vi "HDF5_Init_Disdrometer_Refs.vi"(5 "HDF5 file ref":T2 format="%.0x", 9 "File Exists?":bool, 11 "error in":errorcluster) -> (4 "DisdromRefs":T1 {"Status_dset_deprecated" format="%.0x"; "Spectrum_dset" format="%.0x"; "SpectGroup_ref" format="%.0x"; "HydromType_dset" format="%.0x"; "UnknownVolum_dset" format="%.0x"; "UnknownParticls_dset" format="%.0x"; "NonHydrVolum_dset" format="%.0x"; "NonHydrParticls_dset" format="%.0x"; "ParticlMinDiam_dset" format="%.0x"; "ParticlMaxSpeed_dset" format="%.0x"; "RadarReflect_dset" format="%.0x"; "Visibility_dset" format="%.0x"; "TotalRain_dset" format="%.0x"; "Solid_dset" format="%.0x"; "Liquid_dset" format="%.0x"; "TotalRainRate_dset" format="%.0x"; "TimeStamp_dset" format="%.0x"; "ParticlMinSpeed_dset" format="%.0x"; "MeasdParticles_dset" format="%.0x"; "MaxDiam_dset" format="%.0x"; "BasicGroup_ref" format="%.0x"}, 15 "error out":errorcluster)   [LabVIEW 2018]
doc: "Set up the HDF5 data structure and initialize the references for the Noise1, Noise2, Noise3, and Noise4 Datasets (tables).\n\nData structure:\nNoise1 (Dataset) - 1024 element Double array (waveform) \nNoise2 (Dataset) - 1024 element Double array (waveform) \nNoise3 (Dataset) - 1024 element Double array (waveform) \nNoise4 (Dataset) - 1024 element Double array (waveform)"
uses:
  <vilib>/addons/h5labview2/base/hid_t.ctl
  HDF5_Disdrometer_Refs.ctl
  DisdrometerData.ctl
  DisdromterSummaryData.ctl
  Disdrometer/Disdrometer_Status_Cluster.ctl
  lib_path_mod_20200519.vi
  <vilib>/addons/h5labview2/base/H5Equery.vi
  <vilib>/addons/h5labview2/attrib/H5Awrite.llb/H5Awrite.xnode
  <vilib>/addons/h5labview2/group/H5G.lvlib
  <vilib>/addons/h5labview2/dataset/H5D.lvlib
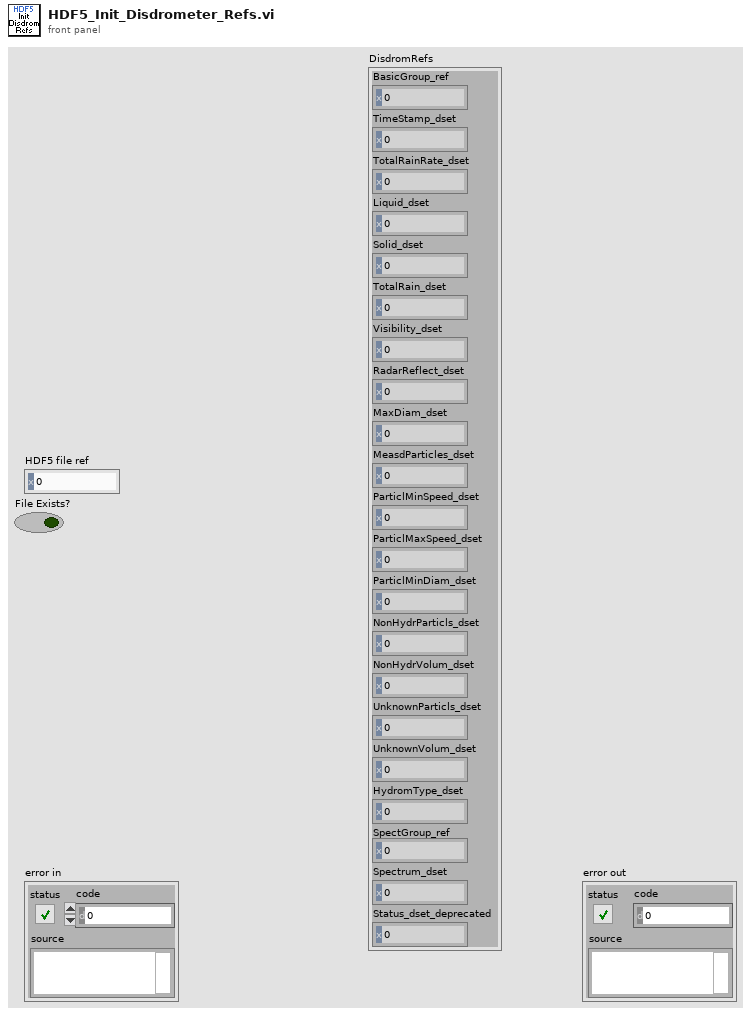
[diagram p1: front panel]
types:
  T1 = typedef "HDF5_Disdrometer_Refs.ctl" = cluster{"BasicGroup_ref":T2, "TimeStamp_dset":T2, "TotalRainRate_dset":T2, "Liquid_dset":T2, "Solid_dset":T2, "TotalRain_dset":T2, "Visibility_dset":T2, "RadarReflect_dset":T2, "MaxDiam_dset":T2, "MeasdParticles_dset":T2, "ParticlMinSpeed_dset":T2, "ParticlMaxSpeed_dset":T2, "ParticlMinDiam_dset":T2, "NonHydrParticls_dset":T2, "NonHydrVolum_dset":T2, "UnknownParticls_dset":T2, "UnknownVolum_dset":T2, "HydromType_dset":T2, "SpectGroup_ref":T2, "Spectrum_dset":T2, "Status_dset_deprecated":T2}
  T2 = typedef "hid_t.ctl" = i32
  T3 = typedef "DisdrometerData.ctl" = cluster{"Spectrum Data":i16[], "DisdromSummary":T4, "Status":T5}
  T4 = typedef "DisdromterSummaryData.ctl" = cluster{"current time":dbl, "Timestamp":dbl, "Total Rain Rate":dbl, "Liquid Rain Rate":dbl, "Solid Rain Rate":dbl, "Total Rainfall":dbl, "Visibility":dbl, "Radar Reflectivity":dbl, "Max Diameter Hail":dbl, "Measured Particles":i32, "Particle Min Speed":i16, "Particle Max Speed":i16, "Particle Min Diam":i16, "NonHydr Particles":i16, "NonHydr Volume":dbl, "Unkn Particles":i16, "Unkn Volume":dbl, "HydroType":i8}
  T5 = typedef "Disdrometer_Status_Cluster.ctl" = cluster{"Laser":bool, "Signal":bool, "LaserTemp_Analog":bool, "LaserTemp_Digital":bool, "LaserCurrent_Analog":bool, "LaserCurrent_Digital":bool, "SensorSupply":bool, "HeatLaserHead":bool, "HeatReceiverHead":bool, "TempSensor":bool, "HeatSupply":bool, "HeatHousing":bool, "HeatHeads":bool, "HeatCarriers":bool, "OutputLaserPower":bool, "Checksum":bool, "StatusInt":u16}
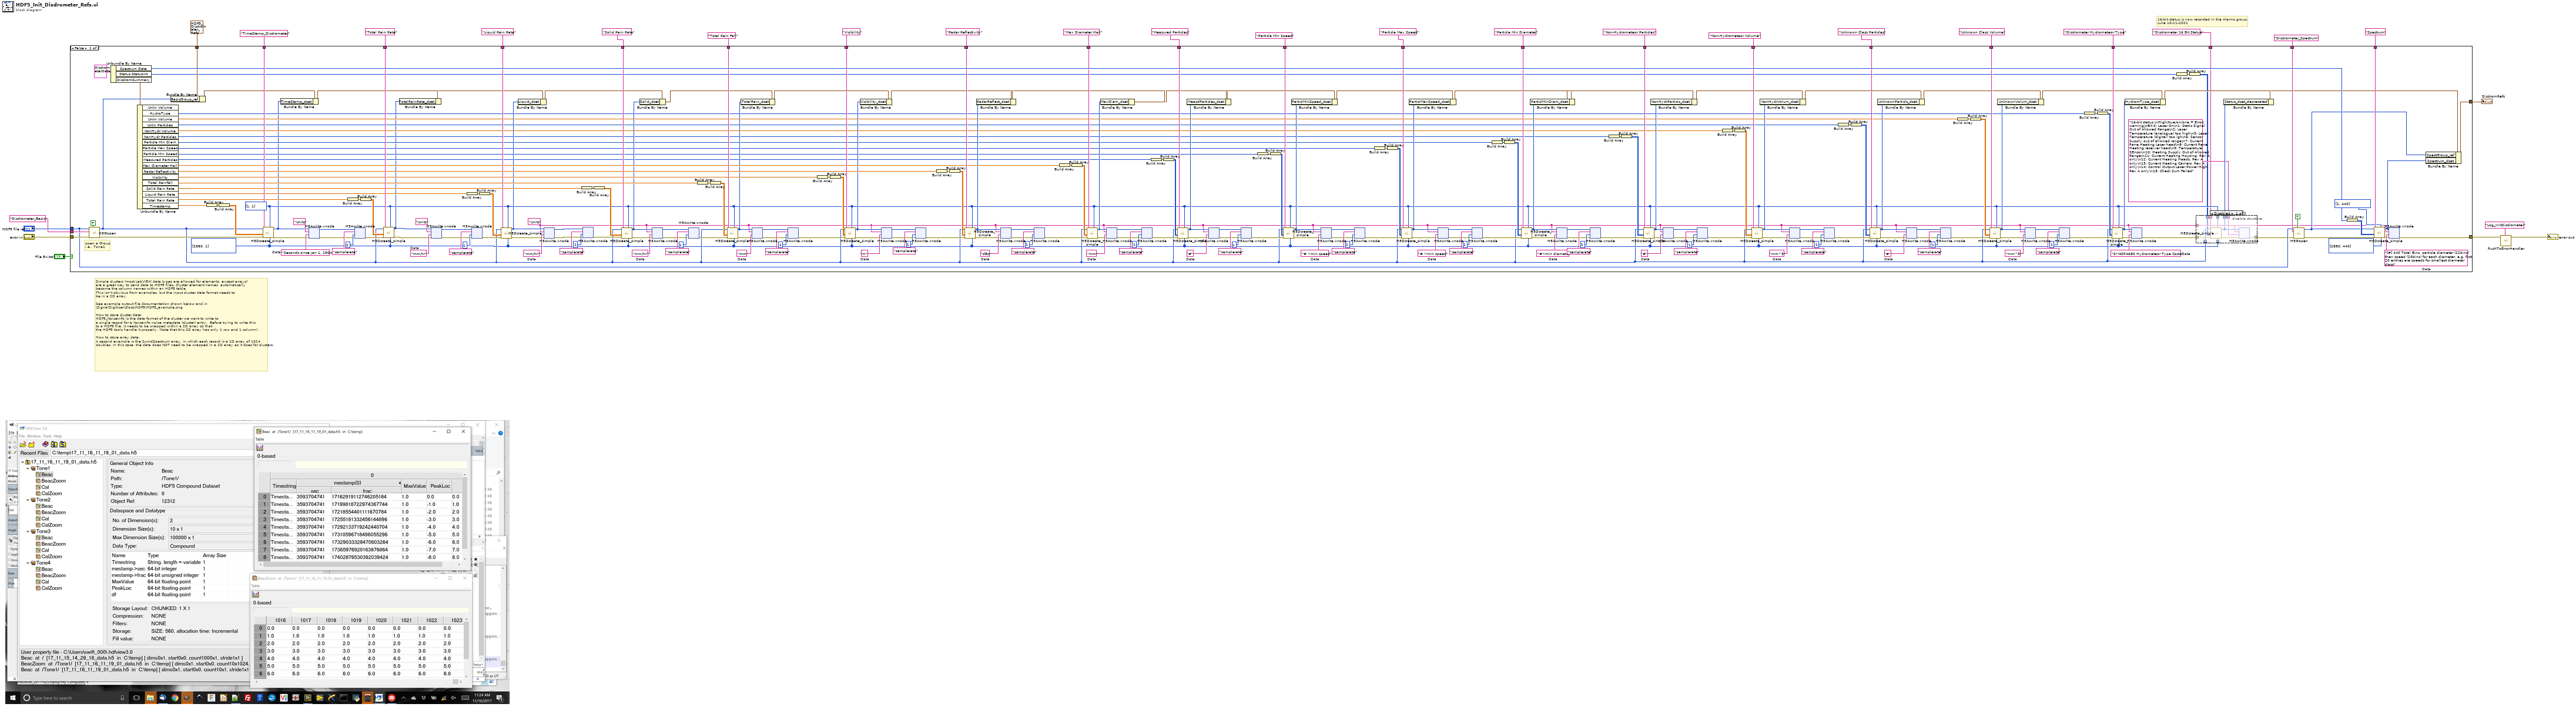
[diagram p0: block diagram]
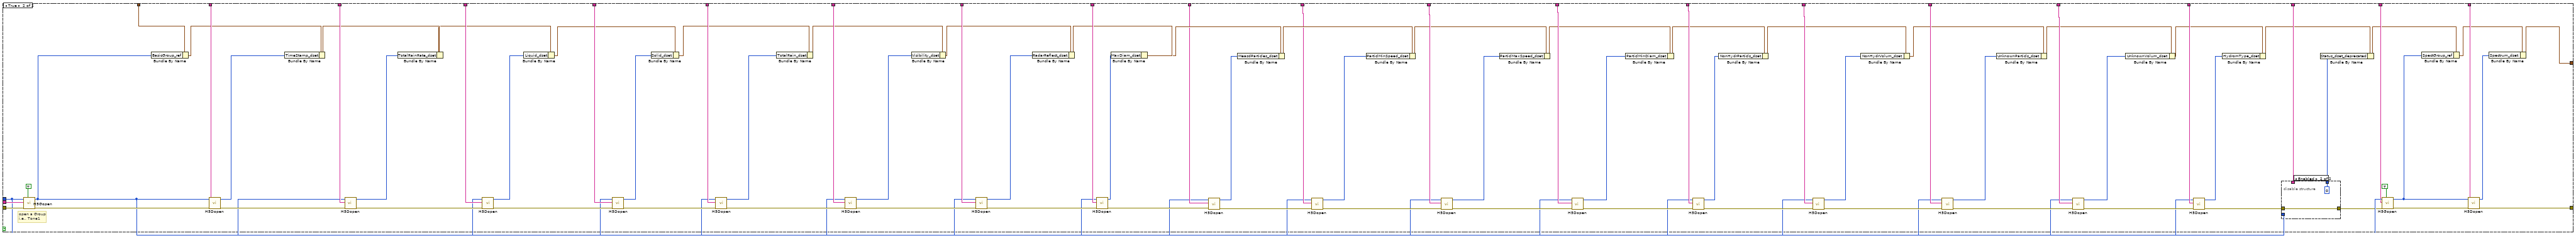
[diagram p3: hidden frame]
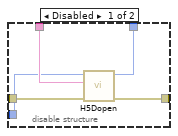
[diagram p4: hidden frame]
diagram:
  # "16-bit status is now recorded in the Alarms group.\nLuke 10-11-2021"
  # "Simple clusters (most LabVIEW data types are allowed for elements, except arrays) \nare a great way to send data to HDF5 files. Cluster element names  automatically\nbecome the column names within an HDF5 table.\nThis isn't obvious from examples, but the input cluster data format needs to \nbe in a 2D array.\n\nSee example output file documentation shown below and in\n\\SignalDigitizer\\Docs\\HDF5\\HDF5_example.png\n\nHow to store cluster data:\nHDF5_NoiseInfo is the data format of the cluster we want to write to \na single record for a NoiseInfo noise metadata (cluster) entry.  Before trying to write this \nto a HDF5 file, it needs to be wrapped within a 2D array so that \nthe HDF5 tools handle it properly. (Note that this 2D array has only 1 row and 1 column).\n\nHow to store array data:\nA second example is the SumdSpectrum array, in which each record is a 1D array of 1024 \ndoubles. In this case, the data does NOT need to be wrapped in a 2D array as it does for clusters."
  n1 = case shown="False" "File Exists?" {
    tunnel: "error in" -> [w283 w1049]
    tunnel: "HDF5 file ref" -> [w178 w1006]
    tunnel: T1 {"BasicGroup_ref"=0, "TimeStamp_dset"=0, "TotalRainRate_dset"=0, "Liquid_dset"=0, "Solid_dset"=0, "TotalRain_dset"=0, "Visibility_dset"=0, "RadarReflect_dset"=0, "MaxDiam_dset"=0, "MeasdParticles_dset"=0, "ParticlMinSpeed_dset"=0, "ParticlMaxSpeed_dset"=0, "ParticlMinDiam_dset"=0, "NonHydrParticls_dset"=0, "NonHydrVolum_dset"=0, "UnknownParticls_dset"=0, "UnknownVolum_dset"=0, "HydromType_dset"=0, "SpectGroup_ref"=0, "Spectrum_dset"=0, "Status_dset_deprecated"=0} ("Cluster") -> [w269 w1029]
    tunnel: "TimeStamp_Disdrometer" ("string") -> [w278 w1046]
    tunnel: "Disdrometer_Basic" ("name") -> [w277 w1045]
    tunnel: [w276 w1010] -> w24
    tunnel: "Spectrum" ("string") -> [w273 w1044]
    tunnel: "Total Rain Rate" ("string") -> [w265 w1037]
    tunnel: "Liquid Rain Rate" ("string") -> [w257 w1038]
    tunnel: "Solid Rain Rate" ("string") -> [w252 w1039]
    tunnel: "Total Rain Fall" ("string") -> [w249 w1040]
    tunnel: "Visibility" ("string") -> [w241 w1041]
    tunnel: "Radar Reflectivity" ("string") -> [w237 w1042]
    tunnel: "Max Diameter Hail" ("string") -> [w232 w1043]
    tunnel: [w213 w1009] -> w4
    tunnel: "Disdrometer_Spectrum" ("name") -> [w211 w1005]
    tunnel: "Measured Particles" ("string") -> [w183 w997]
    tunnel: "Particle Min Speed" ("string") -> [w186 w991]
    tunnel: "Particle Max Speed" ("string") -> [w191 w990]
    tunnel: "Particle Min Diameter" ("string") -> [w194 w989]
    tunnel: "Non-Hydrometeor Particles" ("string") -> [w198 w988]
    tunnel: "Non-Hydrometeor Volume" ("string") -> [w172 w976]
    tunnel: "Unknown Class Particles" ("string") -> [w168 w975]
    tunnel: "Unknown Class Volume" ("string") -> [w165 w974]
    tunnel: "Disdrometer Hydrometeor Type" ("string") -> [w161 w973]
    tunnel: "Disdrometer 16 Bit Status" ("string") -> [w32 w965]
    frame False {
      w138 = "Seconds since Jan 1, 1904"  # Data
      w139 = "mm/hr"  # Data
      w153 = "SYNOP4680 Hydrometeor Type Code"  # Data
      w157 = "mm^3"  # Data
      w158 = "#"  # Data
      w159 = "mm^3"  # Data
      w209 = "#"  # Data
      w203 = "#<min diameter"  # Data
      w202 = "# >min speed"  # Data
      w201 = "# <min speed"  # Data
      w200 = "#"  # Data
      w217 = "[#] 440 Total Bins, particle diameter (22bins) then speed (20bins) for each diameter, e.g. first 20 entries are speeds for smallest diameter class"  # Data
      w218 = "mm"  # Data
      w224 = "dBz"  # Data
      w225 = "m"  # Data
      w226 = "mm"  # Data
      w227 = "mm/hr"  # Data
      w35 = "Units" ("attrib name")
      w230 = "mm/hr"  # Data
      w43 = i32[] [1, 1] ("size(s)")
      w30 = u64[] [2880, 1] ("max size")
      # "open a Group\ni.e., Tone1"
      n2 = call <vilib>:"H5Gopen.vi"("create? (F)"=TRUE, "error in (no error)"=w283, "name"=w277, "ref in"=w178) -> ("error out"=w279:errorcluster, "group out"=w42:T2)  [unwired: 6 in]
      n3 = Unbundle By Name(T3 {"Spectrum Data"=[], "DisdromSummary"={"current time"=0.0, "Timestamp"=0.0, "Total Rain Rate"=0.0, "Liquid Rain Rate"=0.0, "Solid Rain Rate"=0.0, "Total Rainfall"=0.0, "Visibility"=0.0, "Radar Reflectivity"=0.0, "Max Diameter Hail"=0.0, "Measured Particles"=0, "Particle Min Speed"=0, "Particle Max Speed"=0, "Particle Min Diam"=0, "NonHydr Particles"=0, "NonHydr Volume"=0.0, "Unkn Particles"=0, "Unkn Volume"=0.0, "HydroType"=0}, "Status"={"Laser"=TRUE, "Signal"=TRUE, "LaserTemp_Analog"=TRUE, "LaserTemp_Digital"=TRUE, "LaserCurrent_Analog"=TRUE, "LaserCurrent_Digital"=TRUE, "SensorSupply"=TRUE, "HeatLaserHead"=TRUE, "HeatReceiverHead"=TRUE, "TempSensor"=TRUE, "HeatSupply"=TRUE, "HeatHousing"=TRUE, "HeatHeads"=TRUE, "HeatCarriers"=TRUE, "OutputLaserPower"=TRUE, "Checksum"=TRUE, "StatusInt"=0}}) -> ("Spectrum Data"=w272:i16[], "Status.StatusInt"=w31:u16, "DisdromSummary"=w263:T4)
      n4 = Unbundle By Name(w263) -> ("HydroType"=w141:i8, "Unkn Volume"=w142:dbl, "Unkn Particles"=w143:i16, "NonHydr Volume"=w144:dbl, "NonHydr Particles"=w145:i16, "Particle Min Diam"=w146:i16, "Particle Max Speed"=w147:i16, "Particle Min Speed"=w148:i16, "Measured Particles"=w149:i32, "Max Diameter Hail"=w233:dbl, "Radar Reflectivity"=w238:dbl, "Visibility"=w243:dbl, "Total Rainfall"=w248:dbl, "Solid Rain Rate"=w253:dbl, "Liquid Rain Rate"=w258:dbl, "Total Rain Rate"=w261:dbl, "Timestamp"=w262:dbl)  [unwired: 1 out]
      n5 = Bundle By Name(cluster=w269, "BasicGroup_ref"=w42) -> (w268:T1)
      n6 = Build Array(w262) -> (w282:dbl[])
      n7 = Build Array(w282) -> (w281:dbl[][])
      n8 = call <vilib>:"H5Dcreate_simple.vi"("max size"=w30, "chunk size"=w43, "error in (no error)"=w279, "type in"=w281, "name"=w278, "ref in"=w42) -> ("error out"=w136:errorcluster, "dset out"=w133:T2)  [unwired: 4 in]
      n9 = Bundle By Name(cluster=w268, "TimeStamp_dset"=w133) -> (w264:T1)
      n10 = xnode "H5Awrite.xnode"("error in (no error)"=w136, "data"=w138, "attrib name"="Units", "ref in"=w133) -> ("error out"=w121:errorcluster, "ref out"=w119:i32)  [unwired: 3 in, 1 out]
      n11 = Build Array(w261) -> (w266:dbl[])
      n12 = xnode "H5Awrite.xnode"("error in (no error)"=w121, "data"=u32 1, "attrib name"="samplerate", "ref in"=w119) -> ("error out"=w120:errorcluster)  [unwired: 3 in, 2 out]
      n13 = Build Array(w266) -> (w267:dbl[][])
      n14 = call <vilib>:"H5Dcreate_simple.vi"("max size"=w30, "chunk size"=w43, "error in (no error)"=w120, "type in"=w267, "name"=w265, "ref in"=w42) -> ("error out"=w135:errorcluster, "dset out"=w134:T2)  [unwired: 4 in]
      n15 = Bundle By Name(cluster=w264, "TotalRainRate_dset"=w134) -> (w256:T1)
      n16 = xnode "H5Awrite.xnode"("error in (no error)"=w135, "data"=w139, "attrib name"="Units", "ref in"=w134) -> ("error out"=w116:errorcluster, "ref out"=w114:i32)  [unwired: 3 in, 1 out]
      n17 = Build Array(w258) -> (w260:dbl[])
      n18 = xnode "H5Awrite.xnode"("error in (no error)"=w116, "data"=u32 1, "attrib name"="samplerate", "ref in"=w114) -> ("error out"=w115:errorcluster)  [unwired: 3 in, 2 out]
      n19 = Build Array(w260) -> (w259:dbl[][])
      n20 = call <vilib>:"H5Dcreate_simple.vi"("max size"=w30, "chunk size"=w43, "error in (no error)"=w115, "type in"=w259, "name"=w257, "ref in"=w42) -> ("error out"=w229:errorcluster, "dset out"=w228:T2)  [unwired: 4 in]
      n21 = Bundle By Name(cluster=w256, "Liquid_dset"=w228) -> (w247:T1)
      n22 = xnode "H5Awrite.xnode"("error in (no error)"=w229, "data"=w230, "attrib name"=w35, "ref in"=w228) -> ("error out"=w111:errorcluster, "ref out"=w110:i32)  [unwired: 3 in, 1 out]
      n23 = Build Array(w253) -> (w254:dbl[])
      n24 = xnode "H5Awrite.xnode"("error in (no error)"=w111, "data"=u32 1, "attrib name"="samplerate", "ref in"=w110) -> ("error out"=w109:errorcluster)  [unwired: 3 in, 2 out]
      n25 = Build Array(w254) -> (w255:dbl[][])
      n26 = call <vilib>:"H5Dcreate_simple.vi"("max size"=w30, "chunk size"=w43, "error in (no error)"=w109, "type in"=w255, "name"=w252, "ref in"=w42) -> ("error out"=w222:errorcluster, "dset out"=w223:T2)  [unwired: 4 in]
      n27 = Bundle By Name(cluster=w247, "Solid_dset"=w223) -> (w246:T1)
      n28 = xnode "H5Awrite.xnode"("error in (no error)"=w222, "data"=w227, "attrib name"=w35, "ref in"=w223) -> ("error out"=w106:errorcluster, "ref out"=w105:i32)  [unwired: 3 in, 1 out]
      n29 = xnode "H5Awrite.xnode"("error in (no error)"=w106, "data"=u32 1, "attrib name"="samplerate", "ref in"=w105) -> ("error out"=w104:errorcluster)  [unwired: 3 in, 2 out]
      n30 = Build Array(w248) -> (w251:dbl[])
      n31 = Build Array(w251) -> (w250:dbl[][])
      n32 = call <vilib>:"H5Dcreate_simple.vi"("max size"=w30, "chunk size"=w43, "error in (no error)"=w104, "type in"=w250, "name"=w249, "ref in"=w42) -> ("error out"=w129:errorcluster, "dset out"=w221:T2)  [unwired: 4 in]
      n33 = Bundle By Name(cluster=w246, "TotalRain_dset"=w221) -> (w242:T1)
      n34 = xnode "H5Awrite.xnode"("error in (no error)"=w129, "data"=w226, "attrib name"=w35, "ref in"=w221) -> ("error out"=w101:errorcluster, "ref out"=w100:i32)  [unwired: 3 in, 1 out]
      n35 = xnode "H5Awrite.xnode"("error in (no error)"=w101, "data"=u32 1, "attrib name"="samplerate", "ref in"=w100) -> ("error out"=w99:errorcluster)  [unwired: 3 in, 2 out]
      n36 = Build Array(w243) -> (w244:dbl[])
      n37 = Build Array(w244) -> (w245:dbl[][])
      n38 = call <vilib>:"H5Dcreate_simple.vi"("max size"=w30, "chunk size"=w43, "error in (no error)"=w99, "type in"=w245, "name"=w241, "ref in"=w42) -> ("error out"=w130:errorcluster, "dset out"=w220:T2)  [unwired: 4 in]
      n39 = Bundle By Name(cluster=w242, "Visibility_dset"=w220) -> (w236:T1)
      n40 = xnode "H5Awrite.xnode"("error in (no error)"=w130, "data"=w225, "attrib name"=w35, "ref in"=w220) -> ("error out"=w96:errorcluster, "ref out"=w95:i32)  [unwired: 3 in, 1 out]
      n41 = xnode "H5Awrite.xnode"("error in (no error)"=w96, "data"=u32 1, "attrib name"="samplerate", "ref in"=w95) -> ("error out"=w94:errorcluster)  [unwired: 3 in, 2 out]
      n42 = Build Array(w238) -> (w240:dbl[])
      n43 = Build Array(w240) -> (w239:dbl[][])
      n44 = call <vilib>:"H5Dcreate_simple.vi"("max size"=w30, "chunk size"=w43, "error in (no error)"=w94, "type in"=w239, "name"=w237, "ref in"=w42) -> ("error out"=w131:errorcluster, "dset out"=w219:T2)  [unwired: 4 in]
      n45 = Bundle By Name(cluster=w236, "RadarReflect_dset"=w219) -> (w231:T1)
      n46 = xnode "H5Awrite.xnode"("error in (no error)"=w131, "data"=w224, "attrib name"=w35, "ref in"=w219) -> ("error out"=w91:errorcluster, "ref out"=w90:i32)  [unwired: 3 in, 1 out]
      n47 = xnode "H5Awrite.xnode"("error in (no error)"=w91, "data"=u32 1, "attrib name"="samplerate", "ref in"=w90) -> ("error out"=w89:errorcluster)  [unwired: 3 in, 2 out]
      n48 = Build Array(w233) -> (w234:dbl[])
      n49 = Build Array(w234) -> (w235:dbl[][])
      n50 = call <vilib>:"H5Dcreate_simple.vi"("chunk size"=w43, "error in (no error)"=w89, "type in"=w235, "name"=w232, "ref in"=w42) -> ("error out"=w177:errorcluster, "dset out"=w214:T2)  [unwired: 5 in]
      n51 = Bundle By Name(cluster=w231, "MaxDiam_dset"=w214) -> (w180:T1)
      n52 = xnode "H5Awrite.xnode"("error in (no error)"=w177, "data"=w218, "attrib name"=w35, "ref in"=w214) -> ("error out"=w86:errorcluster, "ref out"=w85:i32)  [unwired: 3 in, 1 out]
      n53 = xnode "H5Awrite.xnode"("error in (no error)"=w86, "data"=u32 1, "attrib name"="samplerate", "ref in"=w85) -> ("error out"=w84:errorcluster)  [unwired: 3 in, 2 out]
      n54 = Build Array(w149) -> (w182:i32[])
      n55 = Build Array(w182) -> (w181:i32[][])
      n56 = call <vilib>:"H5Dcreate_simple.vi"("max size"=w30, "chunk size"=w43, "error in (no error)"=w84, "type in"=w181, "name"=w183, "ref in"=w42) -> ("error out"=w205:errorcluster, "dset out"=w204:T2)  [unwired: 4 in]
      n57 = Bundle By Name(cluster=w180, "MeasdParticles_dset"=w204) -> (w187:T1)
      n58 = xnode "H5Awrite.xnode"("error in (no error)"=w205, "data"=w200, "attrib name"=w35, "ref in"=w204) -> ("error out"=w81:errorcluster, "ref out"=w80:i32)  [unwired: 3 in, 1 out]
      n59 = xnode "H5Awrite.xnode"("error in (no error)"=w81, "data"=u32 1, "attrib name"="samplerate", "ref in"=w80) -> ("error out"=w75:errorcluster)  [unwired: 3 in, 2 out]
      n60 = Build Array(w148) -> (w184:i16[])
      n61 = Build Array(w184) -> (w185:i16[][])
      n62 = call <vilib>:"H5Dcreate_simple.vi"("max size"=w30, "chunk size"=w43, "error in (no error)"=w75, "type in"=w185, "name"=w186, "ref in"=w42) -> ("error out"=w132:errorcluster, "dset out"=w206:T2)  [unwired: 4 in]
      n63 = Bundle By Name(cluster=w187, "ParticlMinSpeed_dset"=w206) -> (w190:T1)
      n64 = xnode "H5Awrite.xnode"("error in (no error)"=w132, "data"=w201, "attrib name"=w35, "ref in"=w206) -> ("error out"=w77:errorcluster, "ref out"=w76:i32)  [unwired: 3 in, 1 out]
      n65 = xnode "H5Awrite.xnode"("error in (no error)"=w77, "data"=u32 1, "attrib name"="samplerate", "ref in"=w76) -> ("error out"=w74:errorcluster)  [unwired: 3 in, 2 out]
      n66 = Build Array(w147) -> (w189:i16[])
      n67 = Build Array(w189) -> (w188:i16[][])
      n68 = call <vilib>:"H5Dcreate_simple.vi"("max size"=w30, "chunk size"=w43, "error in (no error)"=w74, "type in"=w188, "name"=w191, "ref in"=w42) -> ("error out"=w124:errorcluster, "dset out"=w207:T2)  [unwired: 4 in]
      n69 = Bundle By Name(cluster=w190, "ParticlMaxSpeed_dset"=w207) -> (w195:T1)
      n70 = xnode "H5Awrite.xnode"("error in (no error)"=w124, "data"=w202, "attrib name"=w35, "ref in"=w207) -> ("error out"=w71:errorcluster, "ref out"=w70:i32)  [unwired: 3 in, 1 out]
      n71 = xnode "H5Awrite.xnode"("error in (no error)"=w71, "data"=u32 1, "attrib name"="samplerate", "ref in"=w70) -> ("error out"=w69:errorcluster)  [unwired: 3 in, 2 out]
      n72 = Build Array(w146) -> (w192:i16[])
      n73 = Build Array(w192) -> (w193:i16[][])
      n74 = call <vilib>:"H5Dcreate_simple.vi"("max size"=w30, "chunk size"=w43, "error in (no error)"=w69, "type in"=w193, "name"=w194, "ref in"=w42) -> ("error out"=w125:errorcluster, "dset out"=w208:T2)  [unwired: 4 in]
      n75 = Bundle By Name(cluster=w195, "ParticlMinDiam_dset"=w208) -> (w199:T1)
      n76 = xnode "H5Awrite.xnode"("error in (no error)"=w125, "data"=w203, "attrib name"=w35, "ref in"=w208) -> ("error out"=w66:errorcluster, "ref out"=w65:i32)  [unwired: 3 in, 1 out]
      n77 = xnode "H5Awrite.xnode"("error in (no error)"=w66, "data"=u32 1, "attrib name"="samplerate", "ref in"=w65) -> ("error out"=w64:errorcluster)  [unwired: 3 in, 2 out]
      n78 = Build Array(w145) -> (w197:i16[])
      n79 = Build Array(w197) -> (w196:i16[][])
      n80 = call <vilib>:"H5Dcreate_simple.vi"("max size"=w30, "chunk size"=w43, "error in (no error)"=w64, "type in"=w196, "name"=w198, "ref in"=w42) -> ("error out"=w176:errorcluster, "dset out"=w210:T2)  [unwired: 4 in]
      n81 = Bundle By Name(cluster=w199, "NonHydrParticls_dset"=w210) -> (w151:T1)
      n82 = xnode "H5Awrite.xnode"("error in (no error)"=w176, "data"=w209, "attrib name"=w35, "ref in"=w210) -> ("error out"=w61:errorcluster, "ref out"=w60:i32)  [unwired: 3 in, 1 out]
      n83 = xnode "H5Awrite.xnode"("error in (no error)"=w61, "data"=u32 1, "attrib name"="samplerate", "ref in"=w60) -> ("error out"=w59:errorcluster)  [unwired: 3 in, 2 out]
      n84 = Build Array(w144) -> (w174:dbl[])
      n85 = Build Array(w174) -> (w173:dbl[][])
      n86 = call <vilib>:"H5Dcreate_simple.vi"("max size"=w30, "chunk size"=w43, "error in (no error)"=w59, "type in"=w173, "name"=w172, "ref in"=w42) -> ("error out"=w126:errorcluster, "dset out"=w156:T2)  [unwired: 4 in]
      n87 = Bundle By Name(cluster=w151, "NonHydrVolum_dset"=w156) -> (w169:T1)
      n88 = xnode "H5Awrite.xnode"("error in (no error)"=w126, "data"=w159, "attrib name"=w35, "ref in"=w156) -> ("error out"=w56:errorcluster, "ref out"=w55:i32)  [unwired: 3 in, 1 out]
      n89 = xnode "H5Awrite.xnode"("error in (no error)"=w56, "data"=u32 1, "attrib name"="samplerate", "ref in"=w55) -> ("error out"=w54:errorcluster)  [unwired: 3 in, 2 out]
      n90 = Build Array(w143) -> (w170:i16[])
      n91 = Build Array(w170) -> (w171:i16[][])
      n92 = call <vilib>:"H5Dcreate_simple.vi"("max size"=w30, "chunk size"=w43, "error in (no error)"=w54, "type in"=w171, "name"=w168, "ref in"=w42) -> ("error out"=w127:errorcluster, "dset out"=w155:T2)  [unwired: 4 in]
      n93 = Bundle By Name(cluster=w169, "UnknownParticls_dset"=w155) -> (w164:T1)
      n94 = xnode "H5Awrite.xnode"("error in (no error)"=w127, "data"=w158, "attrib name"=w35, "ref in"=w155) -> ("error out"=w51:errorcluster, "ref out"=w50:i32)  [unwired: 3 in, 1 out]
      n95 = xnode "H5Awrite.xnode"("error in (no error)"=w51, "data"=u32 1, "attrib name"="samplerate", "ref in"=w50) -> ("error out"=w49:errorcluster)  [unwired: 3 in, 2 out]
      n96 = Build Array(w142) -> (w167:dbl[])
      n97 = Build Array(w167) -> (w166:dbl[][])
      n98 = call <vilib>:"H5Dcreate_simple.vi"("max size"=w30, "chunk size"=w43, "error in (no error)"=w49, "type in"=w166, "name"=w165, "ref in"=w42) -> ("error out"=w128:errorcluster, "dset out"=w154:T2)  [unwired: 4 in]
      n99 = Bundle By Name(cluster=w164, "UnknownVolum_dset"=w154) -> (w160:T1)
      n100 = xnode "H5Awrite.xnode"("error in (no error)"=w128, "data"=w157, "attrib name"=w35, "ref in"=w154) -> ("error out"=w46:errorcluster, "ref out"=w45:i32)  [unwired: 3 in, 1 out]
      n101 = xnode "H5Awrite.xnode"("error in (no error)"=w46, "data"=u32 1, "attrib name"="samplerate", "ref in"=w45) -> ("error out"=w44:errorcluster)  [unwired: 3 in, 2 out]
      n102 = Build Array(w141) -> (w162:i8[])
      n103 = Build Array(w162) -> (w163:i8[][])
      n104 = call <vilib>:"H5Dcreate_simple.vi"("max size"=w30, "chunk size"=w43, "error in (no error)"=w44, "type in"=w163, "name"=w161, "ref in"=w42) -> ("error out"=w175:errorcluster, "dset out"=w152:T2)  [unwired: 4 in]
      n105 = Bundle By Name(cluster=w160, "HydromType_dset"=w152) -> (w39:T1)
      n106 = xnode "H5Awrite.xnode"("error in (no error)"=w175, "data"=w153, "attrib name"=w35, "ref in"=w152) -> ("error out"=w41:errorcluster)  [unwired: 3 in, 2 out]
      n107 = Build Array(w31) -> (w34:u16[])
      n108 = Build Array(w34) -> (w33:u16[][])
      n109 = disable-structure shown="Disabled" {
        disable-tunnel: w43 -> [w294 _]
        disable-tunnel: w42 -> [w293 _]
        disable-tunnel: w41 -> [w292 w314]
        disable-tunnel: [w290 w314] -> w40
        disable-tunnel: [w289 _] -> w37
        disable-tunnel: "16-bit status.\nHigh/true/on/one = Error/warning\nBit 0: Laser On\n1: Static Signal Out of Allowed Range\n2: Laser Temperature (analogue) too high\n3: Laser Temperature (digital) too igh\n6: Sensor Supply out of allowed range\n7: Current Pane Heating Laser head\n8: Current Pane Heating receiver head\n9: Temperature SEnsor\n10: Heating Supply Out of Allowed Range\n11: Current Heating Housing. Rev A only\n12: Current Heating Heads. Rev A only\n13: Current Heating Carriers. Rev A only\n14: Control Output Laser Power High. Rev A only\n15: Check Sum Failed" ("attrib name") -> [w288 _]
        disable-tunnel: w35 -> [w287 _]
        disable-tunnel: w33 -> [w286 _]
        disable-tunnel: w32 -> [w285 _]
        disable-tunnel: w30 -> [w284 _]
        frame Disabled {
          n110 = call <vilib>:"H5Dcreate_simple.vi"("max size"=w284, "chunk size"=w294, "error in (no error)"=w292, "type in"=w286, "name"=w285, "ref in"=w293) -> ("error out"=w291:errorcluster, "dset out"=w289:T2)  [unwired: 4 in]
          n111 = xnode "H5Awrite.xnode"("error in (no error)"=w291, "data"=w288, "attrib name"=w287, "ref in"=w289) -> ("error out"=w290:errorcluster)  [unwired: 3 in, 2 out]
        }
        frame Enabled {
        }
      }
      n112 = Bundle By Name(cluster=w39, "Status_dset_deprecated"=w37) -> (w38:T1)
      n113 = call <vilib>:"H5Gopen.vi"("create? (F)"=TRUE, "error in (no error)"=w40, "name"=w211, "ref in"=w178) -> ("error out"=w150:errorcluster, "group out"=w179:T2)  [unwired: 6 in]
      n114 = Build Array(w272) -> (w274:i16[][])
      n115 = call <vilib>:"H5Dcreate_simple.vi"("max size"=u64[] [2880, 440], "chunk size"=i32[] [1, 440] ("size(s)"), "error in (no error)"=w150, "type in"=w274, "name"=w273, "ref in"=w179) -> ("error out"=w216:errorcluster, "dset out"=w215:T2)  [unwired: 4 in]
      n116 = xnode "H5Awrite.xnode"("error in (no error)"=w216, "data"=w217, "attrib name"=w35, "ref in"=w215) -> ("error out"=w213:errorcluster)  [unwired: 3 in, 2 out]
      n117 = Bundle By Name(cluster=w38, "SpectGroup_ref"=w179, "Spectrum_dset"=w215) -> (w276:T1)
    }
    frame True {
      # "open a Group\ni.e., Tone1"
      n118 = call <vilib>:"H5Gopen.vi"("create? (F)"=TRUE, "error in (no error)"=w1049, "name"=w1045, "ref in"=w1006) -> ("error out"=w1047:errorcluster, "group out"=w964:T2)  [unwired: 6 in]
      n119 = Bundle By Name(cluster=w1029, "BasicGroup_ref"=w964) -> (w1028:T1)
      n120 = call <vilib>:"H5Dopen.vi"("error in (no error)"=w1047, "name"=w1046, "loc in"=w964) -> ("error out"=w1036:errorcluster, "dset out"=w1027:T2)  [unwired: 7 in]
      n121 = Bundle By Name(cluster=w1028, "TimeStamp_dset"=w1027) -> (w1026:T1)
      n122 = call <vilib>:"H5Dopen.vi"("error in (no error)"=w1036, "name"=w1037, "loc in"=w964) -> ("error out"=w1035:errorcluster, "dset out"=w1025:T2)  [unwired: 7 in]
      n123 = Bundle By Name(cluster=w1026, "TotalRainRate_dset"=w1025) -> (w1024:T1)
      n124 = call <vilib>:"H5Dopen.vi"("error in (no error)"=w1035, "name"=w1038, "loc in"=w964) -> ("error out"=w1034:errorcluster, "dset out"=w1023:T2)  [unwired: 7 in]
      n125 = Bundle By Name(cluster=w1024, "Liquid_dset"=w1023) -> (w1022:T1)
      n126 = call <vilib>:"H5Dopen.vi"("error in (no error)"=w1034, "name"=w1039, "loc in"=w964) -> ("error out"=w1033:errorcluster, "dset out"=w1021:T2)  [unwired: 7 in]
      n127 = Bundle By Name(cluster=w1022, "Solid_dset"=w1021) -> (w1020:T1)
      n128 = call <vilib>:"H5Dopen.vi"("error in (no error)"=w1033, "name"=w1040, "loc in"=w964) -> ("error out"=w1032:errorcluster, "dset out"=w1019:T2)  [unwired: 7 in]
      n129 = Bundle By Name(cluster=w1020, "TotalRain_dset"=w1019) -> (w1018:T1)
      n130 = call <vilib>:"H5Dopen.vi"("error in (no error)"=w1032, "name"=w1041, "loc in"=w964) -> ("error out"=w1031:errorcluster, "dset out"=w1017:T2)  [unwired: 7 in]
      n131 = Bundle By Name(cluster=w1018, "Visibility_dset"=w1017) -> (w1016:T1)
      n132 = call <vilib>:"H5Dopen.vi"("error in (no error)"=w1031, "name"=w1042, "loc in"=w964) -> ("error out"=w1030:errorcluster, "dset out"=w1015:T2)  [unwired: 7 in]
      n133 = Bundle By Name(cluster=w1016, "RadarReflect_dset"=w1015) -> (w1014:T1)
      n134 = call <vilib>:"H5Dopen.vi"("error in (no error)"=w1030, "name"=w1043, "loc in"=w964) -> ("error out"=w996:errorcluster, "dset out"=w1013:T2)  [unwired: 7 in]
      n135 = Bundle By Name(cluster=w1014, "MaxDiam_dset"=w1013) -> (w999:T1)
      n136 = call <vilib>:"H5Dopen.vi"("error in (no error)"=w996, "name"=w997, "loc in"=w964) -> ("error out"=w995:errorcluster, "dset out"=w1000:T2)  [unwired: 7 in]
      n137 = Bundle By Name(cluster=w999, "MeasdParticles_dset"=w1000) -> (w998:T1)
      n138 = call <vilib>:"H5Dopen.vi"("error in (no error)"=w995, "name"=w991, "loc in"=w964) -> ("error out"=w994:errorcluster, "dset out"=w1001:T2)  [unwired: 7 in]
      n139 = Bundle By Name(cluster=w998, "ParticlMinSpeed_dset"=w1001) -> (w987:T1)
      n140 = call <vilib>:"H5Dopen.vi"("error in (no error)"=w994, "name"=w990, "loc in"=w964) -> ("error out"=w993:errorcluster, "dset out"=w1002:T2)  [unwired: 7 in]
      n141 = Bundle By Name(cluster=w987, "ParticlMaxSpeed_dset"=w1002) -> (w985:T1)
      n142 = call <vilib>:"H5Dopen.vi"("error in (no error)"=w993, "name"=w989, "loc in"=w964) -> ("error out"=w992:errorcluster, "dset out"=w1003:T2)  [unwired: 7 in]
      n143 = Bundle By Name(cluster=w985, "ParticlMinDiam_dset"=w1003) -> (w986:T1)
      n144 = call <vilib>:"H5Dopen.vi"("error in (no error)"=w992, "name"=w988, "loc in"=w964) -> ("error out"=w977:errorcluster, "dset out"=w1004:T2)  [unwired: 7 in]
      n145 = Bundle By Name(cluster=w986, "NonHydrParticls_dset"=w1004) -> (w972:T1)
      n146 = call <vilib>:"H5Dopen.vi"("error in (no error)"=w977, "name"=w976, "loc in"=w964) -> ("error out"=w982:errorcluster, "dset out"=w981:T2)  [unwired: 7 in]
      n147 = Bundle By Name(cluster=w972, "NonHydrVolum_dset"=w981) -> (w971:T1)
      n148 = call <vilib>:"H5Dopen.vi"("error in (no error)"=w982, "name"=w975, "loc in"=w964) -> ("error out"=w983:errorcluster, "dset out"=w980:T2)  [unwired: 7 in]
      n149 = Bundle By Name(cluster=w971, "UnknownParticls_dset"=w980) -> (w970:T1)
      n150 = call <vilib>:"H5Dopen.vi"("error in (no error)"=w983, "name"=w974, "loc in"=w964) -> ("error out"=w984:errorcluster, "dset out"=w979:T2)  [unwired: 7 in]
      n151 = Bundle By Name(cluster=w970, "UnknownVolum_dset"=w979) -> (w969:T1)
      n152 = call <vilib>:"H5Dopen.vi"("error in (no error)"=w984, "name"=w973, "loc in"=w964) -> ("error out"=w967:errorcluster, "dset out"=w978:T2)  [unwired: 7 in]
      n153 = Bundle By Name(cluster=w969, "HydromType_dset"=w978) -> (w963:T1)
      n154 = disable-structure shown="Enabled" {
        disable-tunnel: w967 -> [w1054 w1056]
        disable-tunnel: [w1053 w1056] -> w966
        disable-tunnel: w965 -> [w1052 _]
        disable-tunnel: w964 -> [w1051 _]
        disable-tunnel: [w1050 T2 0 ("dset out")] -> w961
        frame Disabled {
          n155 = call <vilib>:"H5Dopen.vi"("error in (no error)"=w1054, "name"=w1052, "loc in"=w1051) -> ("error out"=w1053:errorcluster, "dset out"=w1050:T2)  [unwired: 7 in]
        }
        frame Enabled {
        }
      }
      n156 = Bundle By Name(cluster=w963, "Status_dset_deprecated"=w961) -> (w962:T1)
      n157 = call <vilib>:"H5Gopen.vi"("create? (F)"=TRUE, "error in (no error)"=w966, "name"=w1005, "ref in"=w1006) -> ("error out"=w1007:errorcluster, "group out"=w968:T2)  [unwired: 6 in]
      n158 = Bundle By Name(cluster=w962, "SpectGroup_ref"=w968) -> (w1012:T1)
      n159 = call <vilib>:"H5Dopen.vi"("error in (no error)"=w1007, "name"=w1044, "loc in"=w968) -> ("error out"=w1009:errorcluster, "dset out"=w1011:T2)  [unwired: 7 in]
      n160 = Bundle By Name(cluster=w1012, "Spectrum_dset"=w1011) -> (w1010:T1)
    }
  }
  "DisdromRefs" <- w24
  n161 = call "PushToErrorHandler.vi"("ErrorIn"=w4, "ErrorLocation"="Log_InitDisdrometer") -> ("ErrorOut"=→"error out":errorcluster)  [unwired: 5 in]
